vi "Get Current Rotation Raw.vi"(8 "error in":errorcluster, 11 "Gantry in":refnum<class "Gantry.lvclass">) -> (0 "error out":errorcluster, 2 "Current Rotation":dbl, 3 "Gantry out":refnum<class "Gantry.lvclass">)   [LabVIEW 2026, in "Gantry.lvclass"]
uses:
  Gantry.lvclass
  <instrlib>/Aerotech Automation1/Status/TypeDefs/Axis Status Items Cluster.ctl
  <instrlib>/Aerotech Automation1/Status/TypeDefs/Axis Status Item.ctl
  <instrlib>/Aerotech Automation1/Status/Wrappers/Add Axis Status Item.vi
  <instrlib>/Aerotech Automation1/Status/Wrappers/Read Axis Status Item.vi
  FlexWorktable/FlexWorktable.lvclass
  <instrlib>/Aerotech Automation1/Status/Status.lvlib
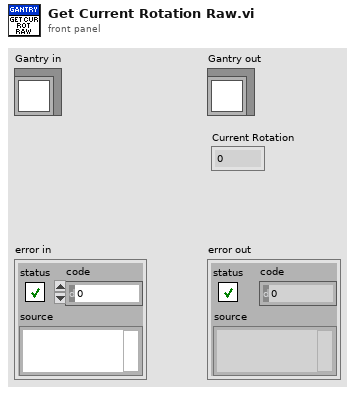
[diagram p1: front panel]
types:
  T1 = typedef "Virtual Modes.ctl" = enum16{"Nonvirtual", "Virtual"}
  T2 = typedef "ControllerDiagPacket.ctl" = cluster{"Number of Diag Packets":i32, "Axes":T3[], "error":errorcluster}
  T3 = typedef "AxisDiagPacket.ctl" = cluster{"Axis Name":string, "Analog Input 0":dbl, "Analog Input 1":dbl, "Axis Fault (num)":i32, "Axis Fault (str)":string, "Axis Fault (bits)":cluster{"AmplifierFault":bool, "AmplifierTemperatureFault":bool, "CcwEndOfTravelLimitFault":bool, "CcwSoftwareLimitFault":bool, "CommunicationLostFault":bool, "CwEndOfTravelLimitFault":bool, "CwSoftwareLimitFault":bool, "EmergencyStopFault":bool, "EncoderFault":bool, "ExternalFault":bool, "FeedbackScalingFault":bool, "GantryMisalignFault ":bool, "HallSensorFault":bool, "InPositionTimeoutFault":bool, "InternalFault":bool, "MarkerSearchFault":bool, "MaxVelocityCommandFault":bool, "MissedInterruptFault":bool, "MotorTemperatureFault":bool, "None":bool, "OverCurrentFault":bool, "PositionErrorFault":bool, "PositionFeedbackFault":bool, "PowerSupplyFault":bool, "ProbeInputFault":bool, "SafeZoneFault":bool, "VelocityErrorFault":bool, "VelocityFeedbackFault":bool, "VoltageClampFault":bool}, "Axis Status (num)":i32, "Axis Status (str)":string, "Axis Status (bits)":cluster{"BacklashActive":bool, "CalibrationEnabled1D":bool, "CalibrationEnabled2D":bool, "CommandValid":bool, "DriveAbortPending":bool, "DrivePending":bool, "Enabling":bool, "GainMappingEnabled":bool, "GantryAligned":bool, "GantryRealigning":bool, "Homed":bool, "Homing":bool, "IFOVEnabled":bool, "JogGenerating":bool, "Jogging":bool, "JoystickControl":bool, "MasterSlaveControl":bool, "MotionBlocked":bool, "MotionClamped":bool, "MoveDone":bool, "None":bool, "NotVirtual":bool, "Profiling":bool, "Stability0":bool, "Stability1":bool, "TrajectoryFiltering":bool, "WaitDone":bool}, "Current Command":sgl, "Current Error":sgl, "Current Feedback":sgl, "Digital Inputs":i32, "Digital Outputs":i32, "Drive Status":i32, "Drive Status (str)":string, "Drive Status (bits)":cluster{"AccelerationPhase":bool, "AutofocusActive":bool, "BrakeOutput":bool, "CcwEndOfTravelLimitInput":bool, "CosineEncoderError":bool, "CurrentClamp":bool, "CwEndOfTravelLimitInput":bool, "DecelerationPhase":bool, "DualLoopActive":bool, "EmergencyStopInput":bool, "Enabled":bool, "EncoderClipping":bool, "GalvoCalibrationEnabled":bool, "GalvoPowerCorrection":bool, "HallAInput":bool, "HallBInput":bool, "HallCInput":bool, "HighResolutionMode":bool, "HomeLimitInput":bool, "InPosition":bool, "InPosition2":bool, "MarkerInput":bool, "MarkerLatch":bool, "MoveActive":bool, "NoMotorSupply":bool, "None":bool, "PowerLimiting":bool, "ProgrammingFlash":bool, "ProgrammingMXH":bool, "PSOHaltLatch":bool, "ServoControl":bool, "SineEncoderError":bool}, "Position Feedback Auxiliary":dbl, "Position Command":dbl, "Position Error":dbl, "Position Feedback":dbl, "Program Position Command":dbl, "Program Position Error":dbl, "Program Position Feedback":dbl, "Velocity Command":dbl, "Velocity Error":dbl, "Velocity Feedback":dbl}
  T4 = typedef "Aerotech Automation1.lvlib/Status.lvlib/Axis Status Items Cluster.ctl" = cluster{"Axis Name":string, "axisStatusItem":T5}
  T5 = typedef "Aerotech Automation1.lvlib/Status.lvlib/Axis Status Item.ctl" = i32
  T6 = typedef "Aerotech Automation1.lvlib/Status.lvlib/Status Refnums.ctl" = cluster{"Status":refnum<k24>, "Status Config":refnum<k24>}
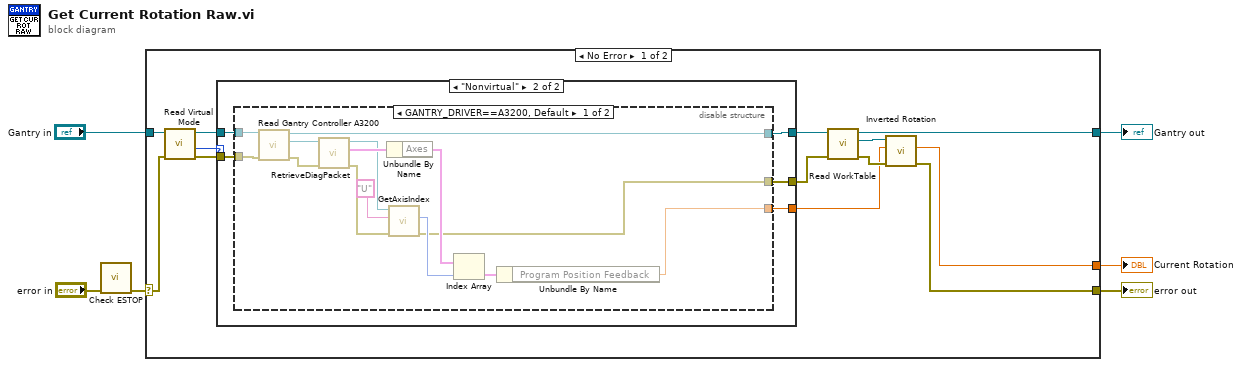
[diagram p0: block diagram]
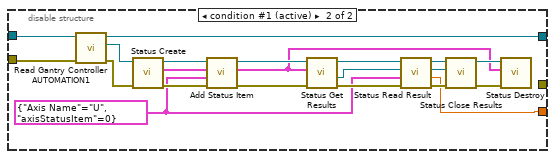
[diagram p3: hidden frame]
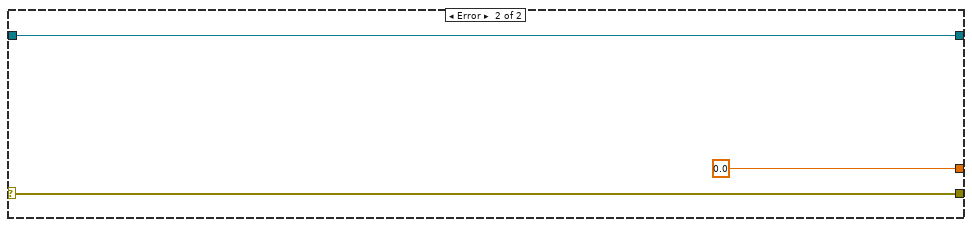
[diagram p4: hidden frame]
diagram:
  n1 = call "Check ESTOP.vi"("error in"="error in") -> ("error out"=w3:errorcluster)  [unwired: 10 in]
  n2 = case shown="No Error" w3 {
    selector: w3 -> [w7 w64]
    tunnel: [w12 w64] -> w6
    tunnel: [w17 w63] -> w5
    tunnel: "Gantry in" -> [w11 w63]
    tunnel: [w13 0.0 ("Program Position Feedback")] -> w1
    frame No Error {
      n3 = call-dynamic "Read Virtual Mode.vi"("error in (no error)"=w7, "Gantry in"=w11) -> ("error out"=w8:errorcluster, "Virtual Mode"=w9:T1, "Gantry out"=w10:refnum<class "Gantry.lvclass">)  [unwired: 6 in, 1 out]
      n4 = case shown="\"Nonvirtual\"" w9 {
        tunnel: w8 -> [w20 w23]
        tunnel: w10 -> [w21 w24]
        tunnel: [w21 w22] -> w16
        tunnel: [_ w26] -> w14
        tunnel: [w20 w25] -> w15
        frame "Virtual" {
        }
        frame "Nonvirtual" {
          n5 = disable-structure shown="GANTRY_DRIVER==A3200, Default" {
            disable-tunnel: [w33 w41] -> w26
            disable-tunnel: [w32 _] -> w25
            disable-tunnel: w24 -> [w31 w44]
            disable-tunnel: w23 -> [w30 w43]
            disable-tunnel: [w27 w42] -> w22
            frame condition #0 {
              n6 = call "Read Gantry Controller A3200.vi"("error in (no error)"=w30, "Gantry in"=w31) -> ("error out"=w29:errorcluster, "A3200 controller out"=w28:refnum<k24>, "Gantry out"=w27:refnum<class "Gantry.lvclass">)  [unwired: 7 in]
              n7 = call "RetrieveDiagPacket.vi"("error in (no error)"=w29, "Controller In"=w28) -> ("error out"=w37:errorcluster, "ControllerDiagPacket"=w40:T2, "Controller Out"=w38:refnum<k24>)  [unwired: 7 in]
              n8 = Unbundle By Name(w40) -> ("Axes"=w39:T3[])
              n9 = call "GetAxisIndex.vi"("error in (no error)"=w37, "axis name"="U", "controller in"=w38) -> ("error out"=w32:errorcluster, "axis index"=w36:i32)  [unwired: 6 in, 1 out]
              n10 = Index Array(array=w39, index=w36) -> (element=w35:T3)
              n11 = Unbundle By Name(w35) -> ("Program Position Feedback"=w33:dbl)
            }
            frame condition #1 (active) {
              w45 = T4 {"Axis Name"="U", "axisStatusItem"=0} ("Axis Status Item")
              n12 = call "Read Gantry Controller AUTOMATION1.vi"("error in (no error)"=w43, "Gantry in"=w44) -> ("error out"=w60:errorcluster, "Controller AUTOMATION1"=w61:refnum<k24>, "Gantry out"=w42:refnum<class "Gantry.lvclass">)  [unwired: 7 in]
              n13 = call <instrlib>:"Status Create.vi"("error in (no error)"=w60, "Controller Refnum"=w61) -> ("error out"=w59:errorcluster, "Status Refnums"=w58:T6, "Controller Refnum out"=w57:refnum<k24>)  [unwired: 7 in]
              n14 = call-poly <instrlib>:"Add Status Item.vi"("error in"=w59, "Axis Status Item"=w45, "Status Refnums"=w58, "Controller Refnum"=w57) -> ("error out"=w55:errorcluster, "Status Refnums out"=w47:T6, "Controller Refnum out"=w56:refnum<k24>)  [unwired: 5 in]
              n15 = call <instrlib>:"Status Get Results.vi"("error in (no error)"=w55, "Status Refnums"=w47, "Controller Refnum"=w56) -> ("error out"=w53:errorcluster, "GetStatusItems"=w52:refnum<k24>, "Controller Refnum out"=w54:refnum<k24>)  [unwired: 5 in, 1 out]
              n16 = call-poly <instrlib>:"Status Read Result.vi"("error in (no error)"=w53, "Axis Status Item"=w45, "Status Results Refnum"=w52, "Controller Refnum"=w54) -> ("error out"=w48:errorcluster, "Data"=w41:dbl, "Status Results Refnum out"=w49:refnum<k24>, "Controller Refnum out"=w51:refnum<k24>)  [unwired: 4 in]
              n17 = call <instrlib>:"Status Close Results.vi"("error in (no error)"=w48, "Status Results Refnum"=w49, "Controller Refnum"=w51) -> ("error out"=w46:errorcluster, "Controller Refnum out"=w50:refnum<k24>)  [unwired: 7 in]
              n18 = call <instrlib>:"Status Destroy.vi"("error in"=w46, "Status Refnums"=w47, "Controller Refnum"=w50) -> ()  [unwired: 7 in, 2 out]
            }
          }
        }
      }
      n19 = call-dynamic "Read WorkTable.vi"("error in"=w15, "Gantry Class in"=w16) -> ("error out"=w18:errorcluster, "Worktable"=w19:refnum<class "FlexWorktable.lvclass">, "Gantry Class out"=w17:refnum<class "Gantry.lvclass">)  [unwired: 7 in]
      n20 = call "Inverted Rotation.vi"("error in (no error)"=w18, "Rotation in"=w14, "FlexWorktable in"=w19) -> ("error out"=w12:errorcluster, "Rotation out"=w13:dbl)  [unwired: 6 in, 1 out]
    }
    frame Error {
    }
  }
  "error out" <- w6
  "Gantry out" <- w5
  "Current Rotation" <- w1
